vi "Frisbee Drive Control.vi"(8 "Circle Info":cluster{dbl, dbl}, 9 "Vertical Constant":dbl=0.5, 10 "Horizontal Constant":dbl=0.9, 11 "Deadband":dbl=0.15) -> (2 "Right Drive":dbl, 3 "Left Drive":dbl)   [LabVIEW 2012]
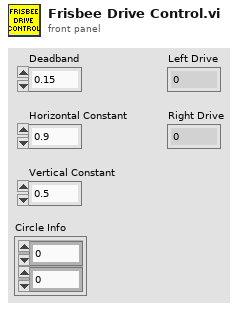
[diagram p1: front panel]
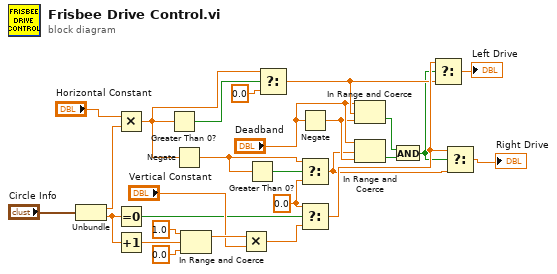
[diagram p0: block diagram]
diagram:
  w2 = 0.0 ("f")
  n1 = Unbundle("Circle Info") -> (w6:dbl, w1:dbl)
  n2 = Multiply(x="Horizontal Constant", y=w6) -> (x*y=w9:dbl)
  n3 = Equal To 0?(x=w1) -> (x = 0?=w4:bool)
  n4 = Increment(x=w1) -> (x+1=w3:dbl)
  n5 = Greater Than 0?(x=w9) -> (x > 0?=w8:bool)
  n6 = Negate(x=w9) -> (-x=w12:dbl)
  n7 = In Range and Coerce(upper limit=1.0, x=w3, lower limit=0.0) -> (coerced(x)=w19:dbl)  [unwired: 1 out]
  n8 = Multiply(x=w19, y="Vertical Constant") -> (x*y=w26:dbl)
  n9 = Greater Than 0?(x=w12) -> (x > 0?=w11:bool)
  n10 = Select(t=w9, s=w8, f=0.0) -> (s? t:f=w25:dbl)
  n11 = Negate(x="Deadband") -> (-x=w23:dbl)
  n12 = Select(t=w12, s=w11, f=w2) -> (s? t:f=w22:dbl)
  n13 = Select(t=w2, s=w4, f=w26) -> (s? t:f=w27:dbl)
  n14 = In Range and Coerce(upper limit="Deadband", x=w25, lower limit=w23) -> (In Range?=w20:bool)  [unwired: 1 out]
  n15 = In Range and Coerce(upper limit="Deadband", x=w22, lower limit=w23) -> (In Range?=w21:bool)  [unwired: 1 out]
  n16 = And(x=w20, y=w21) -> (x .and. y?=w13:bool)
  n17 = Select(t=w27, s=w13, f=w25) -> (s? t:f=→"Left Drive":dbl)
  n18 = Select(t=w27, s=w13, f=w22) -> (s? t:f=→"Right Drive":dbl)
